vi "Unregister panel from running.vi"(8 "error in (no error)":errorcluster, 11 "Fiber Auto Collimation panel in":refnum<class "Fiber Auto Collimation panel.lvclass">) -> (0 "error out":errorcluster, 3 "Fiber Auto Collimation panel out":refnum<class "Fiber Auto Collimation panel.lvclass">)   [LabVIEW 2018, in "Fiber Auto Collimation panel.lvclass"]
doc: "Registers a Panel as no longer being \"running\". Should only be called on the Panel VI itself, never externally. It should be called once at the start of the panel and then never again (unless the panel stops and restarts, of course).\n\nIn the interest of speed and simplicity, any entries in the list of running panels matching the same class and the same clone name are removed. If done properly this should remove one entry and leave the rest. If this isn't working, add checks to your specific impementation to generate an error if zero, or two or more entries are removed.\n\nThis VI also removes the panel from any SubPanel it might be embedded inside of.\n\nThis VI attempts to run regardless of any input errors."
uses:
  Fiber Auto Collimation panel.lvclass
  Fiber Auto Collimation panel.lvclass/Fiber Auto Collimation panel.ctl
  <vilib>/Utility/error.llb/Clear Errors.vi
  <vilib>/Utility/LVClass/Get LV Class Name.vi
  <userlib>/nLight Error Handling/Log any errors.vi
  <userlib>/nLight Error Handling/Merge errors no loss.vi
  References/Fiber Auto Collimation References.lvclass
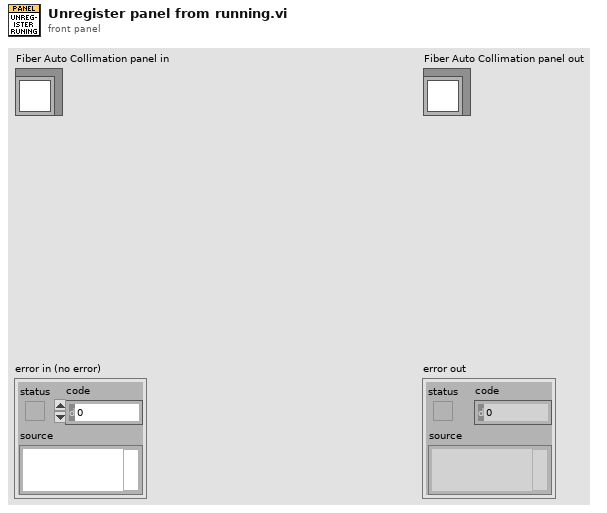
[diagram p1: front panel]
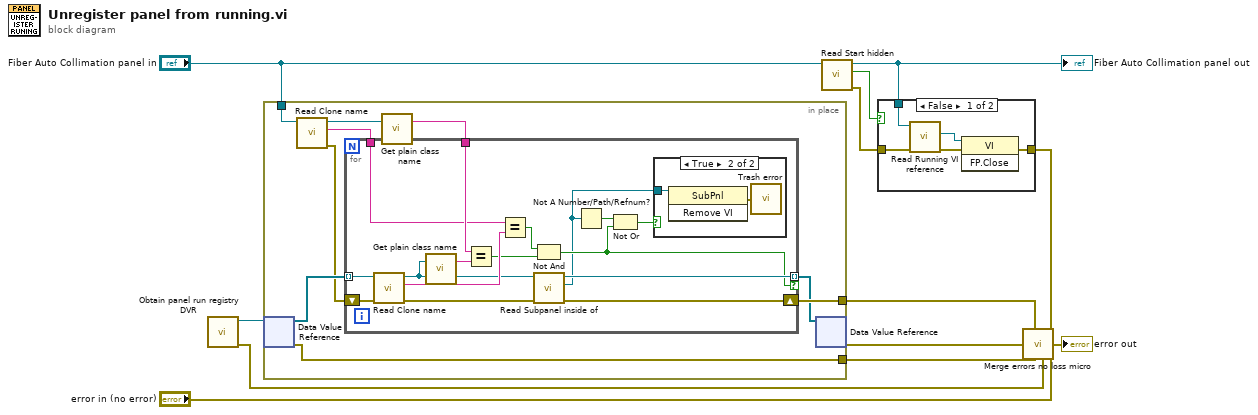
[diagram p0: block diagram]
diagram:
  n1 = call "Obtain panel run registry DVR.vi"() -> ("error out"=w9:errorcluster, "Panel registration DVR"=w12:refnum<data-value>)  [unwired: 10 in]
  n2 = in-place {
    in-place-border: "Fiber Auto Collimation panel in" -> [w19]
    in-place-border: [w21] -> w10
    in-place-border: [w16] -> w3
    n3 = in-place-dvr #1(w12) -> (w20:refnum<class "Fiber Auto Collimation panel.lvclass">[], w21:errorcluster)
    n4 = call "Read Clone name.vi"("Fiber Auto Collimation panel in"=w19) -> ("error out"=w17:errorcluster, "Clone name"=w14:string, "Fiber Auto Collimation panel out"=w18:refnum<class "Fiber Auto Collimation panel.lvclass">)  [unwired: 8 in]
    n5 = call <userlib>:"Get plain class name.vi"("Any class"=w18) -> ("Plain class name"=w15:string)  [unwired: 2 in]
    n6 = for {
      tunnel: w20 -> [w37] mode=indexing
      tunnel: [w26] -> w13 mode=indexing if=w24
      shift-right: [w27] -> w16
      shift-left: w17 -> [w36]
      tunnel: w15 -> [w34]
      tunnel: w14 -> [w32]
      n7 = call "Read Clone name.vi"("error in (no error)"=w36, "Fiber Auto Collimation panel in"=w37) -> ("error out"=w29:errorcluster, "Clone name"=w33:string, "Fiber Auto Collimation panel out"=w28:refnum<class "Fiber Auto Collimation panel.lvclass">)  [unwired: 7 in]
      n8 = call <userlib>:"Get plain class name.vi"("Any class"=w28) -> ("Plain class name"=w35:string)  [unwired: 2 in]
      n9 = Equal?(x=w34, y=w35) -> (x = y?=w31:bool)
      n10 = Equal?(x=w32, y=w33) -> (x = y?=w30:bool)
      n11 = Not And(1:w31, 2:w30) -> (0:w24:bool)
      n12 = call "Read Subpanel inside of.vi"("error in (no error)"=w29, "Fiber Auto Collimation panel in"=w28) -> ("error out"=w27:errorcluster, "Subpanel inside of"=w22:refnum<vi>, "Fiber Auto Collimation panel out"=w26:refnum<class "Fiber Auto Collimation panel.lvclass">)  [unwired: 7 in]
      n13 = Not A Number/Path/Refnum?(number/path/refnum=w22) -> (NaN/Path/Refnum?=w25:bool)
      n14 = Not Or(1:w24, 2:w25) -> (0:w23:bool)
      n15 = case shown="True" w23 {
        tunnel: w22 -> [_ w39]
        frame False {
        }
        frame True {
          n16 = invoke class="SubPnl" method="Remove VI"(reference=w39) -> (error out=w38:errorcluster)  [unwired: 2 in, 2 out]
          n17 = call <userlib>:"Trash error.vi"("error in"=w38) -> ()  [unwired: 15 in]
        }
      }
    }
    n18 = in-place-dvr #1(w13) -> (w11:errorcluster)  [unwired: 1 out]
  }
  n19 = call "Read Start hidden.vi"("Fiber Auto Collimation panel in"="Fiber Auto Collimation panel in") -> ("error out"=w4:errorcluster, "Start hidden"=w6:bool, "Fiber Auto Collimation panel out"=w5:refnum<class "Fiber Auto Collimation panel.lvclass">)  [unwired: 8 in]
  "Fiber Auto Collimation panel out" <- w5
  n20 = case shown="False" w6 {
    tunnel: w5 -> [w44 _]
    tunnel: w4 -> [w41 w45]
    tunnel: [w40 w45] -> w2
    frame False {
      n21 = call "Read Running VI reference.vi"("error in (no error)"=w41, "Fiber Auto Collimation panel in"=w44) -> ("error out"=w43:errorcluster, "Running VI reference"=w42:refnum<vi>)  [unwired: 7 in, 1 out]
      n22 = invoke class="VI" method="FP.Close"(reference=w42, error in=w43) -> (error out=w40:errorcluster)  [unwired: 1 in, 2 out]
    }
    frame True {
    }
  }
  n23 = call <userlib>:"Merge errors no loss micro.vi"("error in (no error) 2"=w3, "error in (no error) 1"=w11, "error in (no error) 5"=w10, "error in (no error) 4"=w2, "error in (no error) 6"=w9, "error in (no error) 7"="error in (no error)") -> ("error out"=→"error out":errorcluster)  [unwired: 3 in]
